vi "auto_ir_test.vi"() -> ()   [LabVIEW 2012, in "Mecanum Drive.lvrbt"]
uses:
  Mecanum Drive.lvrbt
  SubVIs/State_Typ.ctl
  <vilib>/NXT/HiTechnic/HiTechnic Controls/HiTechnic Port.ctl
  <vilib>/NXT/Block Support/NXT_InputPort.ctl
  SubVIs/auto_drive_TYP.ctl
  <vilib>/NXT/Hardware/Plugins/Tetrix DC Motor/TetrixDCMotorAddress.ctl
  <vilib>/NXT/Hardware/Plugins/Tetrix 180 deg Servo/Tetrix180ServoAddress.ctl
  <vilib>/NXT/Dual Mode Library/Display/drawNumber.vi
  <vilib>/NXT/Dual Mode Library/Waits/Wait_Num.vi
  <vilib>/NXT/NXTIO Xnodes/NXTIONodeSubVIs/TETRIX IO Check Battery.vi
  <vilib>/NXT/Dual Mode Library/Waits/Wait_Num(msec).vi
  <vilib>/NXT/NXTIO Xnodes/NXTIONodeSubVIs/TETRIX IO Reset Encoders.vi
  <vilib>/NXT/NXTIO Xnodes/NXTIONodeSubVIs/TETRIX IO Move Servos.vi
  <vilib>/NXT/NXTIO Xnodes/NXTIONodeSubVIs/TETRIX IO Motor Status.vi
  <vilib>/NXT/Dual Mode Library/Sound/Tone.vi
  <vilib>/NXT/NXTIO Xnodes/NXTIONodeSubVIs/TETRIX IO Stop DC Motors.vi
  <vilib>/NXT/Subs/LVHSConnector.ctl
  <vilib>/NXT/NXTIO Xnodes/AddressXNode/NXTIOAddress.xnode
  <vilib>/NXT/NXTIO Xnodes/NXTIOXNode/NXTIO.xnode
  <vilib>/NXT/LegoClasses/BrickReference/BrickReference.lvclass
panel:
  out "Enabled":bool
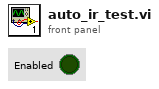
[diagram p1: front panel]
types:
  T1 = typedef "auto_drive_TYP.ctl" = cluster{"Left Y":i8, "Right Y":i8, "Power (100)":i8, "Wait (ms)":u32, "Enc/Deg Target":i32, "Move Type":enum16{"Relative Degrees", "Wait", "Encoder"}}
  T2 = typedef "State_Typ.ctl" = enum16{"Stop", "Check for Position 3", "Check for Position 2", "Move", "Reset Enc", "Read Enc"}
  T3 = typedef "HiTechnic Port.ctl" = cluster{"Port":T4, "MUX Port":u8}
  T4 = typedef "NXT_InputPort.ctl" = u32
  T5 = typedef "TetrixDCMotorAddress.ctl" = i32
  T6 = typedef "LVHSConnector.ctl" = refnum<class "BrickReference.lvclass">
  T7 = typedef "Tetrix180ServoAddress.ctl" = i32
  T8 = cluster{"TetrixDCMotor":T5, "TetrixDCMotor 2":T5}
  T9 = cluster{"Direction (0-9)":i16, "Signal Strength (Array)":u8[]}
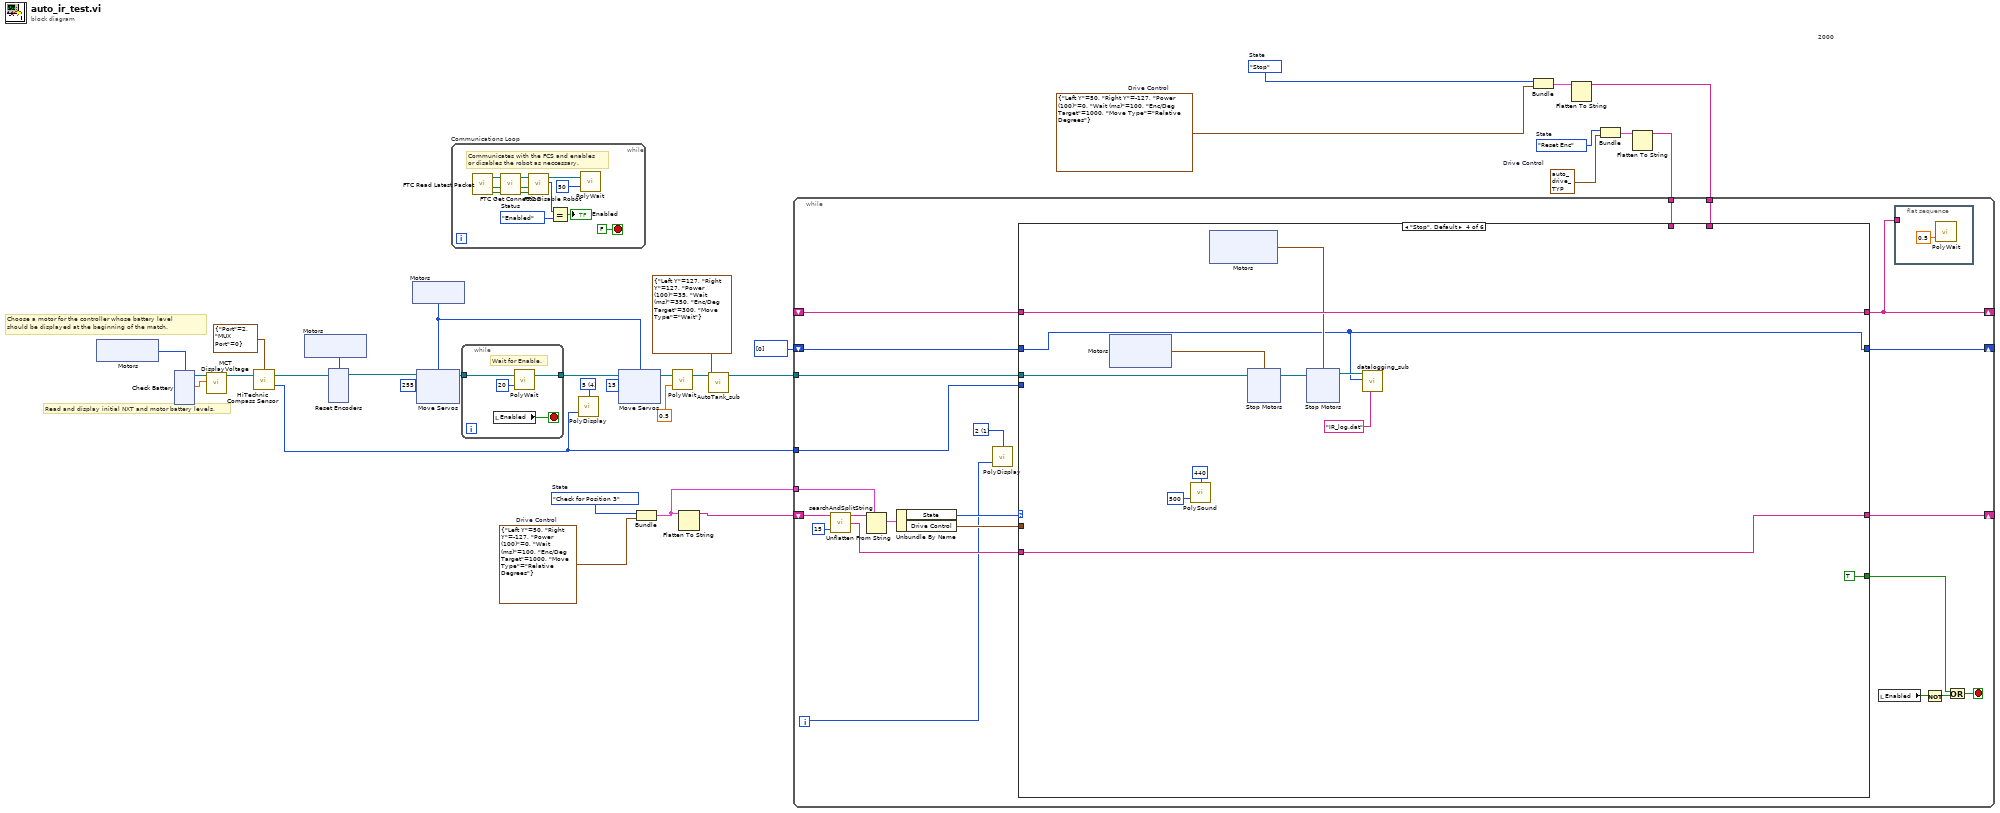
[diagram p0: block diagram]
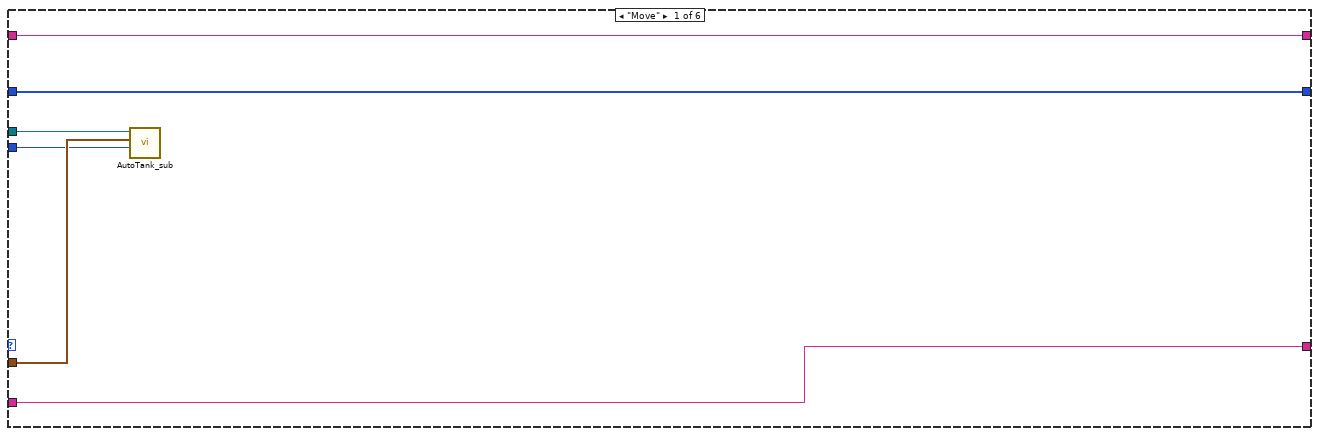
[diagram p2: hidden frame]
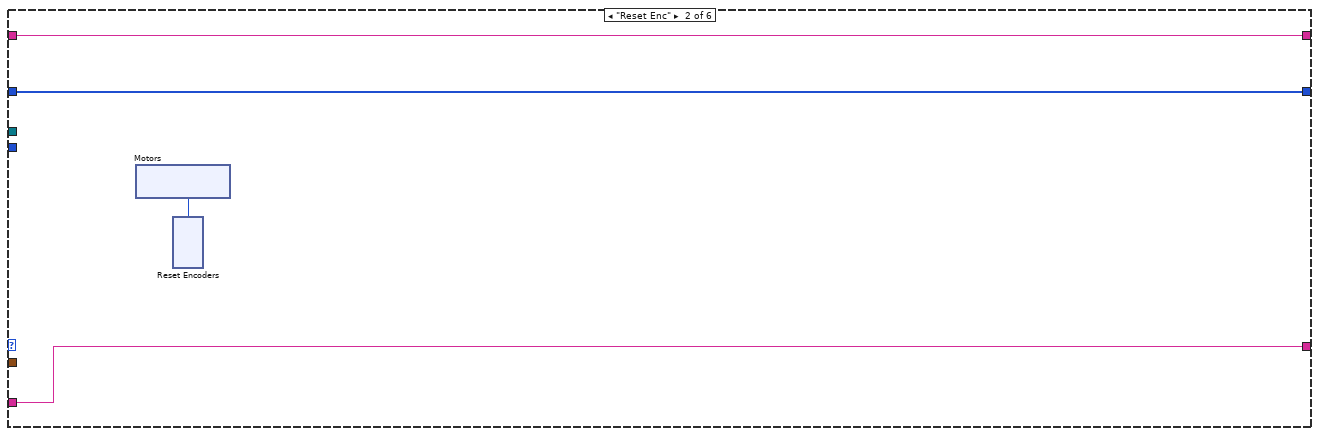
[diagram p3: hidden frame]
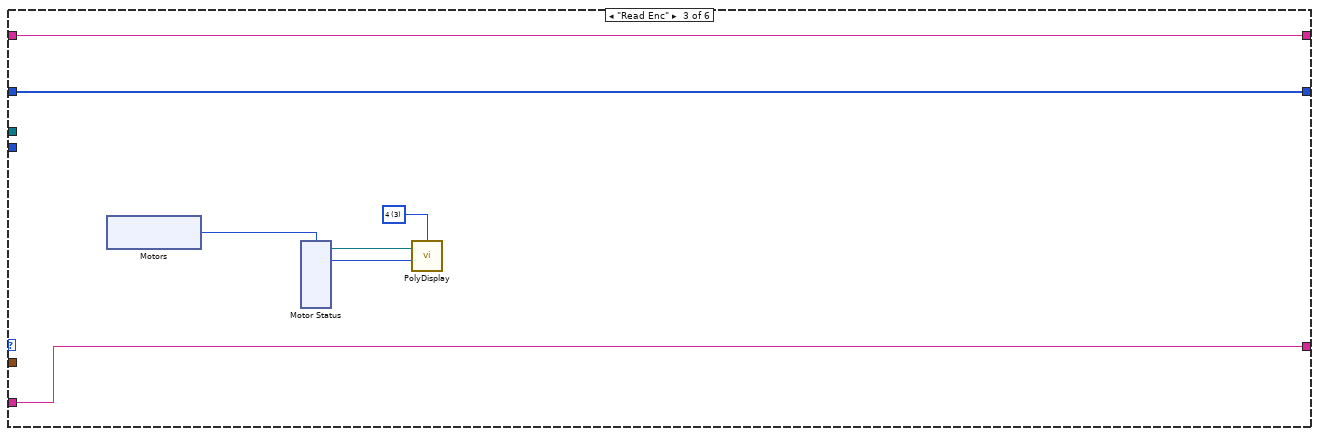
[diagram p4: hidden frame]
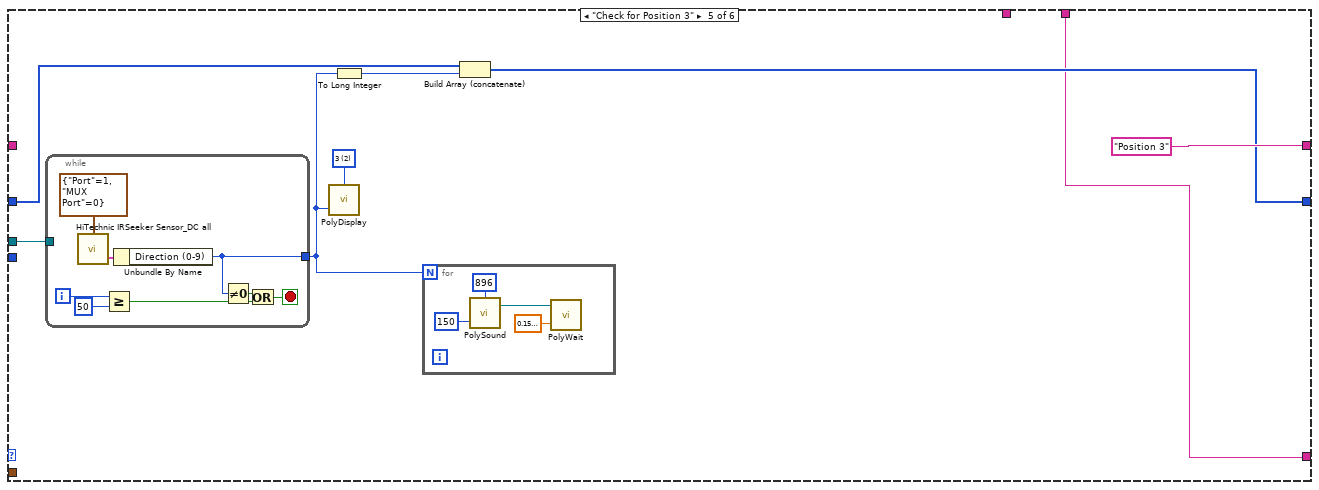
[diagram p5: hidden frame]
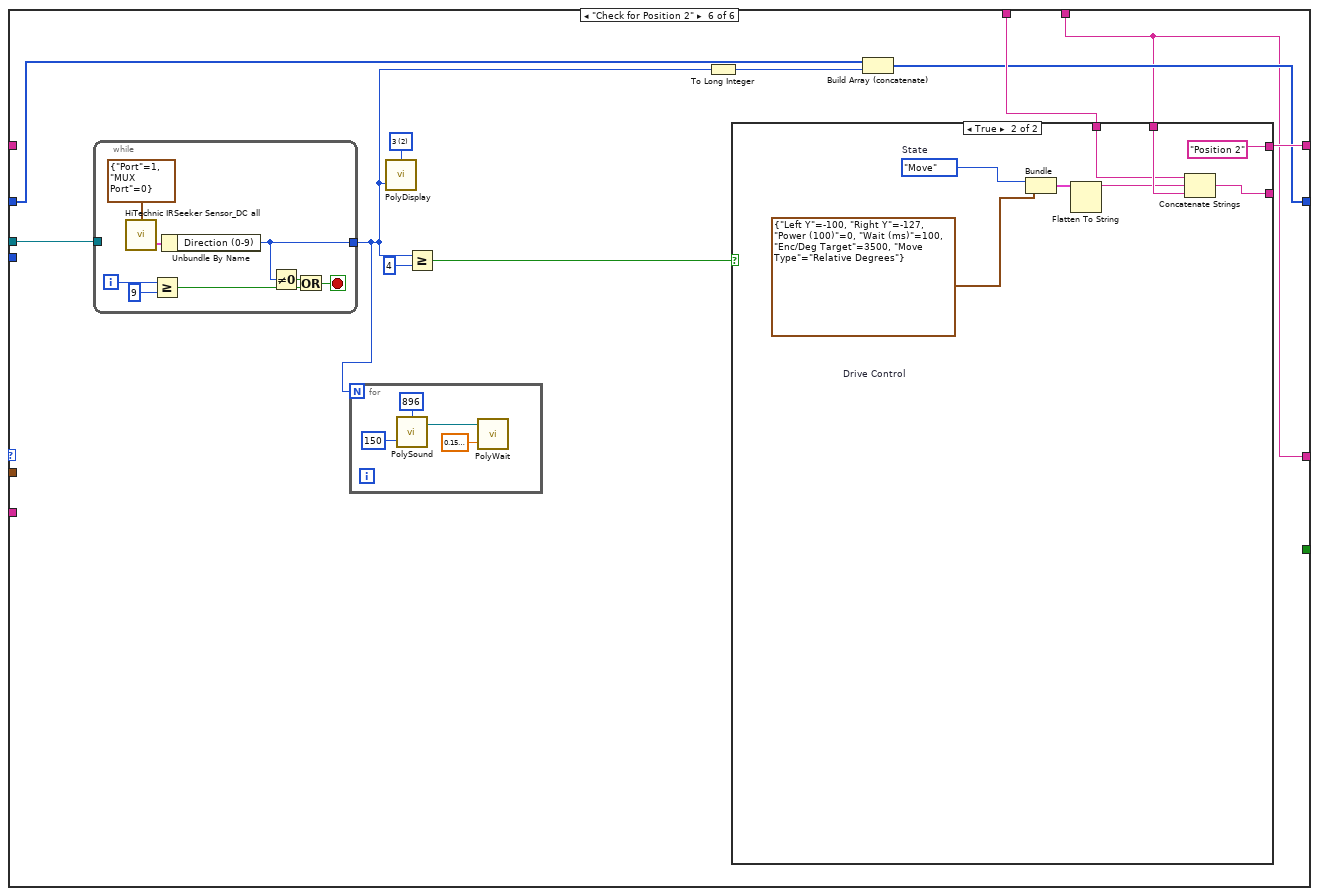
[diagram p6: hidden frame]
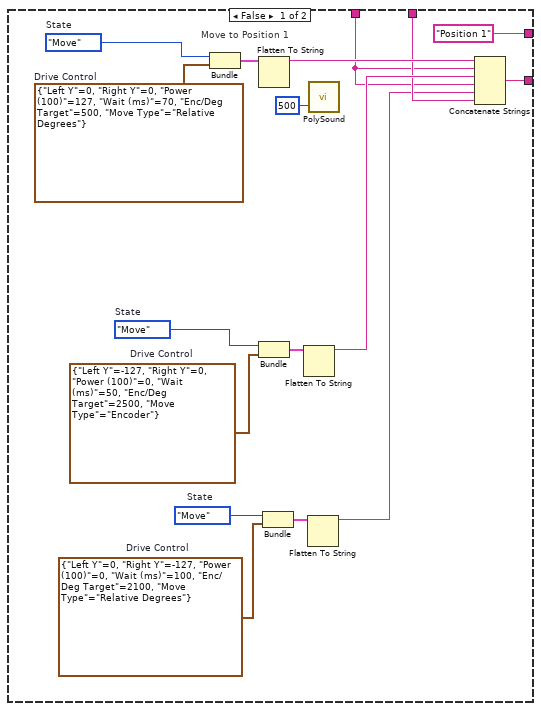
[diagram p7: hidden frame]
diagram:
  w15 = T1 {"Left Y"=0, "Right Y"=0, "Power (100)"=0, "Wait (ms)"=0, "Enc/Deg Target"=0, "Move Type"=enum."Relative Degrees"}  # Drive Control
  w17 = State_Typ."Reset Enc"  # State
  w22 = T1 {"Left Y"=50, "Right Y"=-127, "Power (100)"=0, "Wait (ms)"=100, "Enc/Deg Target"=1000, "Move Type"=enum."Relative Degrees"}  # Drive Control
  w23 = State_Typ."Stop"  # State
  w26 = i16 4 items=["1", "2", "3", "4", "5", "6", "7", "8", "9", "10", "11", "12"] ("Line")
  w33 = T1 {"Left Y"=50, "Right Y"=-127, "Power (100)"=0, "Wait (ms)"=100, "Enc/Deg Target"=1000, "Move Type"=enum."Relative Degrees"}  # Drive Control
  w32 = State_Typ."Check for Position 3"  # State
  # "2000"
  # "Read and display initial NXT and motor battery levels."
  # "Choose a motor for the controller whose battery level \nshould be displayed at the beginning of the match."
  n1 = xnode "Motors"() -> ("Motor"=w29:T5)
  n2 = xnode "Check Battery"("Motors"=w29) -> ("Voltage 1"=w30:sgl, "NXT/EV3"=w31:T6)  [unwired: 1 in]
  n3 = call <vilib>:"MCT DisplayVoltage.vi"("Motor Voltage"=w30, "NXT"=w31) -> ("NXT"=w27:T6)  [unwired: 9 in]
  n4 = call <vilib>:"HiTechnic Compass Sensor.vi"("NXT/EV3"=w27, "Port/MUX"=T3 {"Port"=2, "MUX Port"=0}) -> ("Heading (degrees)"=w25:i16, "NXT/EV3"=w4:T6)  [unwired: 1 in]
  n5 = xnode "Motors"() -> ("Motor"=w5:T5)
  n6 = xnode "Reset Encoders"("Motors"=w5, "NXT/EV3"=w4) -> ("NXT/EV3"=w3:T6)
  n7 = xnode "Motors"() -> ("Motor"=w11:T7)
  n8 = xnode "Move Servos"("Position 1"=u8 255, "Motors"=w11, "NXT/EV3"=w3) -> ("NXT/EV3"=w14:T6)
  n9 = while "Communications Loop" {
    stop <- FALSE stop-if-true
    # "Communicates with the FCS and enables \nor disables the robot as neccessary."
    n10 = call <vilib>:"FTC Read Latest Packet.vi"() -> ("Packet Received?"=w43:bool, "Stopped?"=w42:bool, "NXT"=w45:T6)  [unwired: 6 in, 3 out]
    n11 = call <vilib>:"FTC Get Connection Status.vi"("Packet Received?"=w43, "Stopped?"=w42, "NXT"=w45) -> ("Online?"=w34:bool, "Stopped?"=w35:bool, "NXT"=w44:T6)  [unwired: 5 in]
    n12 = call <vilib>:"FTC Disable Robot.vi"("Online?"=w34, "Stopped?"=w35, "NXT"=w44) -> ("Enabled?"=w38:enum16{"Disabled", "Enabled"}, "NXT"=w40:T6)  [unwired: 3 in]
    n13 = Equal?(x=w38, y=enum16{"Disabled", "Enabled"}."Enabled") -> (x = y?=→"Enabled":bool)
    n14 = call-poly <vilib>:"PolyWait.vi"("Time (100 msec)"=u32 50 ("Time (msec)"), "NXT/EV3"=w40) -> ()  [unwired: 2 in, 1 out]
  }
  n15 = while {
    tunnel: [w47] -> w10
    tunnel: w14 -> [w46]
    stop <- w48 stop-if-true
    # "Wait for Enable."
    n16 = local read "Enabled"() -> (w48:bool)
    n17 = call-poly <vilib>:"PolyWait.vi"("Time (100 msec)"=u32 20 ("Time (msec)"), "NXT/EV3"=w46) -> ("NXT/EV3"=w47:T6)  [unwired: 2 in]
  }
  n18 = call-poly <vilib>:"PolyDisplay.vi"("number"=w25, "Line"=w26) -> ()  [unwired: 2 in, 1 out]
  n19 = xnode "Move Servos"("Position 1"=u8 15, "Motors"=w11, "NXT/EV3"=w10) -> ("NXT/EV3"=w7:T6)
  n20 = Bundle("State"=w32, "Drive Control"=w33) -> (w1:cluster{"State":T2, "Drive Control":T1})  [unwired: 1 in]
  n21 = call-poly <vilib>:"PolyWait.vi"("Time (1 sec)"=sgl 0.5, "NXT/EV3"=w7) -> ("NXT/EV3"=w8:T6)  [unwired: 2 in]
  n22 = Flatten To String(anything=w1) -> (data string=w2:string)  [unwired: 3 in, 2 out]
  n23 = call "AutoTank_sub.vi"("Drive Control"=T1 {"Left Y"=127, "Right Y"=127, "Power (100)"=35, "Wait (ms)"=350, "Enc/Deg Target"=300, "Move Type"=enum."Wait"}, "NXT/EV3"=w8) -> ("NXT/EV3 out"=w12:T6)  [unwired: 8 in, 1 out]
  n24 = Bundle("State"=w23, "Drive Control"=w22) -> (w24:cluster{"State":T2, "Drive Control":T1})  [unwired: 1 in]
  n25 = Flatten To String(anything=w24) -> (data string=w21:string)  [unwired: 3 in, 2 out]
  n26 = Bundle("State"=w17, "Drive Control"=w15) -> (w18:cluster{"State":T2, "Drive Control":T1})  [unwired: 1 in]
  n27 = Flatten To String(anything=w18) -> (data string=w16:string)  [unwired: 3 in, 2 out]
  n28 = while {
    tunnel: w12 -> [w72]
    shift-right: [w63] -> _
    shift-left: w2 -> [w61]
    tunnel: w1 -> [w64]
    shift-right: [w54] -> _
    shift-left: _ -> [w62]
    tunnel: w21 -> [w59]
    tunnel: w25 -> [w53]
    shift-right: [w52] -> _
    shift-left: i32[] [0] -> [w51]
    tunnel: w16 -> [w50]
    i -> [w55]
    stop <- w71 stop-if-true
    w56 = i16 1 items=["1", "2", "3", "4", "5", "6", "7", "8", "9", "10", "11", "12"] ("Line")
    n29 = call <vilib>:"searchAndSplitString.vi"("offset (0)"=15 ("length (rest)"), "string"=w61) -> ("match + rest of string"=w60:string, "substring before match"=w66:string)  [unwired: 1 in, 1 out]
    n30 = Unflatten From String(type=w64, binary string=w66) -> (value=w65:cluster{"State":T2, "Drive Control":T1})  [unwired: 3 in, 2 out]
    n31 = Unbundle By Name(w65) -> ("State"=w57:T2, "Drive Control"=w67:T1)
    n32 = call-poly <vilib>:"PolyDisplay.vi"("number"=w55, "Line"=w56) -> ()  [unwired: 2 in, 1 out]
    n33 = case shown="\"Stop\", Default" w57 {
      tunnel: w72 -> [w79 _ _ w116 w131 w154]
      tunnel: [_ _ _ TRUE _ _] -> w70
      tunnel: w67 -> [w78 _ _ _ _ _]
      tunnel: w60 -> [w77 w83 w95 w114 _ _]
      tunnel: [w77 w83 w95 w114 w129 w149] -> w63
      tunnel: [w76 w82 w94 w113 "Position 3" w159] -> w54
      tunnel: w62 -> [w76 w82 w94 w113 _ _]
      tunnel: w59 -> [_ _ _ _ w129 w149]
      tunnel: w53 -> [w75 _ _ _ _ _]
      tunnel: [w74 w80 w89 w108 w133 w157] -> w52
      tunnel: w51 -> [w74 w80 w89 w108 w134 w156]
      tunnel: w50 -> [_ _ _ _ _ w158]
      frame "Move" {
        n34 = call "AutoTank_sub.vi"("Target Heading (Degrees)"=w75, "Drive Control"=w78, "NXT/EV3"=w79) -> ()  [unwired: 7 in, 2 out]
      }
      frame "Reset Enc" {
        n35 = xnode "Motors"() -> ("Motor"=w81:T5)
        n36 = xnode "Reset Encoders"("Motors"=w81) -> ()  [unwired: 1 in, 1 out]
      }
      frame "Read Enc" {
        w91 = i16 3 items=["1", "2", "3", "4", "5", "6", "7", "8", "9", "10", "11", "12"] ("Line")
        n37 = xnode "Motors"() -> ("Motor"=w93:T5)
        n38 = xnode "Motor Status"("Motors"=w93) -> ("Position 1"=w92:i32, "NXT/EV3"=w90:T6)  [unwired: 1 in, 1 out]
        n39 = call-poly <vilib>:"PolyDisplay.vi"("number"=w92, "NXT/EV3"=w90, "Line"=w91) -> ()  [unwired: 1 in, 1 out]
      }
      frame "Stop", Default {
        n40 = xnode "Motors"() -> ("Motor"=w112:cluster{"TetrixDCMotor":T5, "TetrixDCMotor":T5})
        n41 = call-poly <vilib>:"PolySound.vi"("Duration (500 ms)"=u16 500, "Tone (440 Hz)"=u16 440) -> ()  [unwired: 2 in, 1 out]
        n42 = xnode "Motors"() -> ("Motor"=w111:cluster{"TetrixDCMotor":T5, "TetrixDCMotor":T5})
        n43 = xnode "Stop Motors"("Motors"=w112, "NXT/EV3"=w116) -> ("NXT/EV3"=w110:T6)
        n44 = xnode "Stop Motors"("Motors"=w111, "NXT/EV3"=w110) -> ("NXT/EV3"=w109:T6)
        n45 = call "datalogging_sub.vi"("Filename"="IR_log.dat", "Encoder Vals"=w108, "NXT/EV3 In"=w109) -> ()  [unwired: 8 in, 1 out]
      }
      frame "Check for Position 3" {
        w135 = i16 2 items=["1", "2", "3", "4", "5", "6", "7", "8", "9", "10", "11", "12"] ("Line")
        n46 = while {
          tunnel: w131 -> [_]
          tunnel: [w146] -> w130
          i -> [w144]
          stop <- w141 stop-if-true
          n47 = call <vilib>:"HiTechnic IRSeeker Sensor_DC all.vi"("Port/MUX"=T3 {"Port"=1, "MUX Port"=0}) -> ("All Info"=w148:T9)  [unwired: 2 in, 1 out]
          n48 = Greater Or Equal?(x=w144, y=50 ("x")) -> (x >= y?=w142:bool)
          n49 = Unbundle By Name(w148) -> ("Direction (0-9)"=w146:i16)
          n50 = Not Equal To 0?(x=w146) -> (x != 0?=w145:bool)
          n51 = Or(x=w145, y=w142) -> (x .or. y?=w141:bool)
        }
        n52 = call-poly <vilib>:"PolyDisplay.vi"("number"=w130, "Line"=w135) -> ()  [unwired: 2 in, 1 out]
        n53 = To Long Integer(number=w130) -> (32bit integer=w132:i32)
        n54 = for {
          N: w130 -> [_]
          n55 = call-poly <vilib>:"PolySound.vi"("Duration (500 ms)"=u16 150, "Tone (440 Hz)"=u16 896) -> ("NXT/EV3"=w138:T6)  [unwired: 2 in]
          n56 = call-poly <vilib>:"PolyWait.vi"("Time (1 sec)"=sgl 0.15, "NXT/EV3"=w138) -> ()  [unwired: 2 in, 1 out]
        }
        n57 = Build Array (concatenate)(w134, w132) -> (w133:i32[])
      }
      frame "Check for Position 2" {
        w152 = i16 2 items=["1", "2", "3", "4", "5", "6", "7", "8", "9", "10", "11", "12"] ("Line")
        n58 = while {
          tunnel: [w169] -> w150
          tunnel: w154 -> [_]
          i -> [w167]
          stop <- w164 stop-if-true
          n59 = call <vilib>:"HiTechnic IRSeeker Sensor_DC all.vi"("Port/MUX"=T3 {"Port"=1, "MUX Port"=0}) -> ("All Info"=w171:T9)  [unwired: 2 in, 1 out]
          n60 = Greater Or Equal?(x=w167, y=9 ("x")) -> (x >= y?=w165:bool)
          n61 = Unbundle By Name(w171) -> ("Direction (0-9)"=w169:i16)
          n62 = Not Equal To 0?(x=w169) -> (x != 0?=w168:bool)
          n63 = Or(x=w168, y=w165) -> (x .or. y?=w164:bool)
        }
        n64 = for {
          N: w150 -> [_]
          n65 = call-poly <vilib>:"PolySound.vi"("Duration (500 ms)"=u16 150, "Tone (440 Hz)"=u16 896) -> ("NXT/EV3"=w161:T6)  [unwired: 2 in]
          n66 = call-poly <vilib>:"PolyWait.vi"("Time (1 sec)"=sgl 0.15, "NXT/EV3"=w161) -> ()  [unwired: 2 in, 1 out]
        }
        n67 = call-poly <vilib>:"PolyDisplay.vi"("number"=w150, "Line"=w152) -> ()  [unwired: 2 in, 1 out]
        n68 = Greater Or Equal?(x=w150, y=i16 4) -> (x >= y?=w151:bool)
        n69 = To Long Integer(number=w150) -> (32bit integer=w155:i32)
        n70 = case shown="True" w151 {
          tunnel: [w185 w193] -> _
          tunnel: ["Position 1" "Position 2"] -> w159
          tunnel: w149 -> [w177 w191]
          tunnel: w158 -> [w172 w189]
          frame False {
            w175 = T1 {"Left Y"=0, "Right Y"=-127, "Power (100)"=0, "Wait (ms)"=100, "Enc/Deg Target"=2100, "Move Type"=enum."Relative Degrees"}  # Drive Control
            w176 = State_Typ."Move"  # State
            w183 = T1 {"Left Y"=-127, "Right Y"=0, "Power (100)"=0, "Wait (ms)"=50, "Enc/Deg Target"=2500, "Move Type"=enum."Encoder"}  # Drive Control
            w184 = State_Typ."Move"  # State
            w187 = T1 {"Left Y"=0, "Right Y"=0, "Power (100)"=127, "Wait (ms)"=70, "Enc/Deg Target"=500, "Move Type"=enum."Relative Degrees"}  # Drive Control
            w188 = State_Typ."Move"  # State
            # "Move to Position 1"
            n71 = Bundle("State"=w188, "Drive Control"=w187) -> (w186:cluster{"State":T2, "Drive Control":T1})  [unwired: 1 in]
            n72 = Flatten To String(anything=w186) -> (data string=w179:string)  [unwired: 3 in, 2 out]
            n73 = Bundle("State"=w184, "Drive Control"=w183) -> (w182:cluster{"State":T2, "Drive Control":T1})  [unwired: 1 in]
            n74 = Bundle("State"=w176, "Drive Control"=w175) -> (w174:cluster{"State":T2, "Drive Control":T1})  [unwired: 1 in]
            n75 = Flatten To String(anything=w182) -> (data string=w181:string)  [unwired: 3 in, 2 out]
            n76 = Flatten To String(anything=w174) -> (data string=w173:string)  [unwired: 3 in, 2 out]
            n77 = call-poly <vilib>:"PolySound.vi"("Duration (500 ms)"=u16 500) -> ()  [unwired: 3 in, 1 out]
            n78 = Concatenate Strings(w179, w172, w181, w172, w173, w177) -> (w185:string)
          }
          frame True {
            w195 = T1 {"Left Y"=-100, "Right Y"=-127, "Power (100)"=0, "Wait (ms)"=100, "Enc/Deg Target"=3500, "Move Type"=enum."Relative Degrees"}  # Drive Control
            w194 = State_Typ."Move"  # State
            n79 = Bundle("State"=w194, "Drive Control"=w195) -> (w196:cluster{"State":T2, "Drive Control":T1})  [unwired: 1 in]
            n80 = Flatten To String(anything=w196) -> (data string=w190:string)  [unwired: 3 in, 2 out]
            n81 = Concatenate Strings(w189, w190, w191) -> (w193:string)
          }
        }
        n82 = Build Array (concatenate)(w156, w155) -> (w157:i32[])
      }
    }
    n83 = local read "Enabled"() -> (w69:bool)
    n84 = flat-sequence {
      tunnel: w54 -> [_]
      frame #0 {
        n85 = call-poly <vilib>:"PolyWait.vi"("Time (1 sec)"=sgl 0.5) -> ()  [unwired: 3 in, 1 out]
      }
    }
    n86 = Not(x=w69) -> (.not. x?=w58:bool)
    n87 = Or(x=w70, y=w58) -> (x .or. y?=w71:bool)
  }
